vi "ToString.vi"(8 "error in (no error)":errorcluster, 11 "IsType in":refnum<class "IsType.lvclass">) -> (0 "error out":errorcluster, 2 "String":string, 3 "IsType out":refnum<class "IsType.lvclass">)   [LabVIEW 2017, in "Constraint.lvlib" / "IsType.lvclass"]
doc: "Returns a string representation of the object."
uses:
  IsType.lvclass
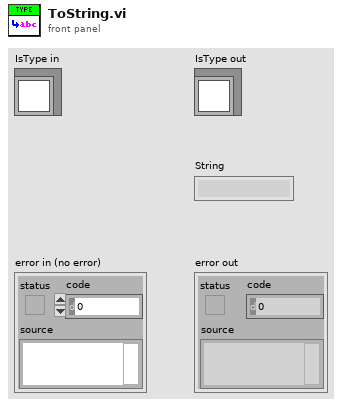
[diagram p1: front panel]
types:
  T1 = typedef "NI_Data Type.lvlib/Data Type.ctl" = enum8{"Invalid Type", "Void", "I8", "I16", "I32", "I64", "U8", "U16", "U32", "U64", "Single Float", "Double Float", "Extended Float", "Single Complex", "Double Complex", "Extended Complex", "Enum U8", "Enum U16", "Enum U32", "Enum U64", "Single Float With Unit", "Double Float With Unit", "Extended Float With Unit", "Single Complex with Unit", "Double Complex with Unit", "Extended Complex with Unit", "Boolean", "String", "Path", "Picture", "Tag", "Array", "Cluster", "Variant", "LV Variant", "Waveform", "Timestamp", "Digital Waveform", "Digital Data", "ExpressData", "Refnum", "External Data", "VI", "Poly VI", "LabVIEW Class Instance", "Fixed Point", "Set Collection", "Map Collection"}
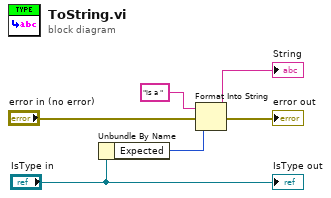
[diagram p0: block diagram]
diagram:
  n1 = Unbundle By Name("IsType in") -> ("Expected"=w2:T1)
  n2 = Format Into String(initial string="is a ", error in="error in (no error)", w2) -> (resulting string=→"String":string, error out=→"error out":errorcluster)  [unwired: 1 in]
  "IsType out" <- "IsType in"
